vi "inverse kinematics for 4R robot.vi"(5 "y":dbl, 7 "x":dbl) -> (1 "theta3":dbl=-1.5707963267948966, 2 "theta2":dbl=2.186276035465284, 3 "theta1":dbl=0.4776583090622547)   [LabVIEW 2014]
doc: "Inverse Kinematics for the 3R planar subsystem of the 4R robot.\n\nDetermines joint angles required to place the end effector at the desired (x,y) position."
panel:
  in  "L3":dbl=4.0
  in  "L2":dbl=4.0
  in  "L1":dbl=4.0
  # "Assuming that the desired coordinates are of the form (x,y,theta), the joint angle theta0=theta.\nThis VI calculates values for theta1, theta2, theta3 that will put the end effector at the desired\ncoordinates (x,y)."
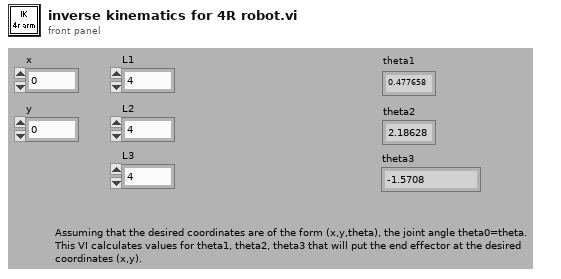
[diagram p1: front panel]
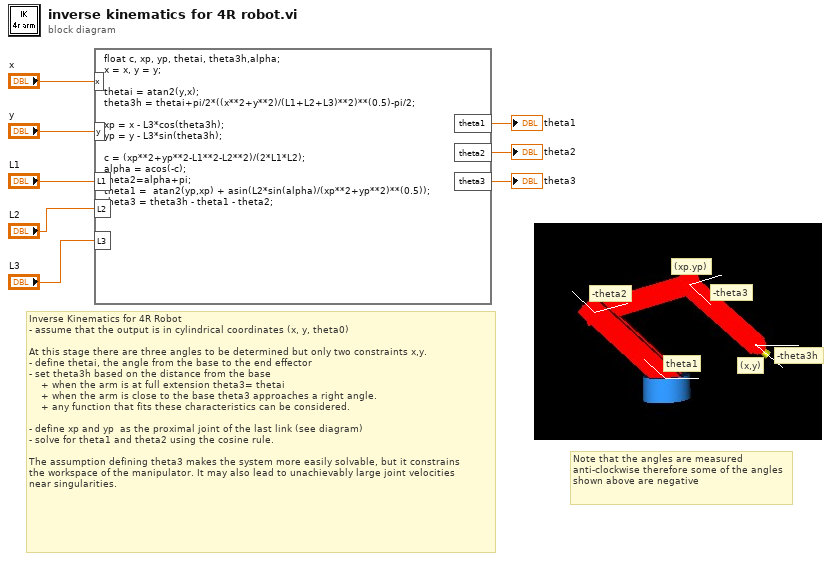
[diagram p0: block diagram]
diagram:
  # "(x,y)"
  # "(xp.yp)"
  # "-theta3h"
  # "Note that the angles are measured anti-clockwise therefore some of the angles shown above are negative"
  # "-theta3"
  # "-theta2"
  # "theta1"
  # "Inverse Kinematics for 4R Robot\n- assume that the output is in cylindrical coordinates (x, y, theta0)\n\nAt this stage there are three angles to be determined but only two constraints x,y.\n- define thetai, the angle from the base to the end effector\n- set theta3h based on the distance from the base\n    + when the arm is at full extension theta3= thetai\n    + when the arm is close to the base theta3 approaches a right angle. \n    + any function that fits these characteristics can be considered.\n\n- define xp and yp  as the proximal joint of the last link (see diagram)\n- solve for theta1 and theta2 using the cosine rule.\n\nThe assumption defining theta3 makes the system more easily solvable, but it constrains\nthe workspace of the manipulator. It may also lead to unachievably large joint velocities\nnear singularities."
  n1 = formula code="float c, xp, yp, thetai, theta3h,alpha;\nx = x, y = y;\n\nthetai = atan2(y,x);\ntheta3h = thetai+pi/2*((x**2+y**2)/(L1+L2+L3)**2)**(0.5)-pi/2;\n\nxp = x - L3*cos(theta3h);\nyp = y - L3*sin(theta3h);\n\nc = (xp**2+yp**2-L1**2-L2**2)/(2*L1*L2);\nalpha = acos(-c);\ntheta2=alpha+pi;\ntheta1 =  atan2(yp,xp) + asin(L2*sin(alpha)/(xp**2+yp**2)**(0.5));\ntheta3 = theta3h - theta1 - theta2;"("x"="x", "y"="y", "L1"="L1", "L2"="L2", "L3"="L3") -> ("theta1"=→"theta1":dbl, "theta2"=→"theta2":dbl, "theta3"=→"theta3":dbl)
